vi "TAT-Create Reciepe.vi"(8 "Error In":errorcluster) -> (0 "error out":errorcluster)   [LabVIEW 2017]
uses:
  Controls/Recipe.ctl
  <vilib>/Utility/config.llb/Write Key (String).vi
  <vilib>/Utility/config.llb/Read Key (String).vi
  <vilib>/Utility/config.llb/NI_LVConfig.lvlib
panel:
  in  "Lable Data":T1
  in  "Reference Barcode":T2
  in  "T-Bin Seq. Select":T3 {"First" max=8 step=1; "Second" max=8 step=1; "Third" max=8 step=1; "Fourth" max=8 step=1; "Fifth" max=8 step=1; "Gun Enable" max=8}
  in  "Torquing Station Sensor Selection":T4
  in  "A-Bin Seq. Select":T5 {"Camera-2 Trig" max=8 step=1; "Camera-1 Trig" max=8 step=1; "First" max=8 step=1; "Second" max=8 step=1; "Third" max=8 step=1; "Fourth" max=8 step=1; "Fifth" max=8 step=1; "Sixth" max=8; "Seventh" max=8; "Eighth" max=8}
  in  "Ass. Sensor Select":T6 {"Gun \nProg. no." max=8 step=1; "Camera-2\n Prog. no." max=8 step=1; "Camera-1\n Prog. no." max=8 step=1}
  in  "Delete":bool
  in  "Save":bool
  in  "BACK":bool
  in  "PART NAME":string(combo)
  # "TEST PARAMETER SETTING"
  # "Bin No."
  # "Bin No."
  # "Bin No."
  # "Bin No."
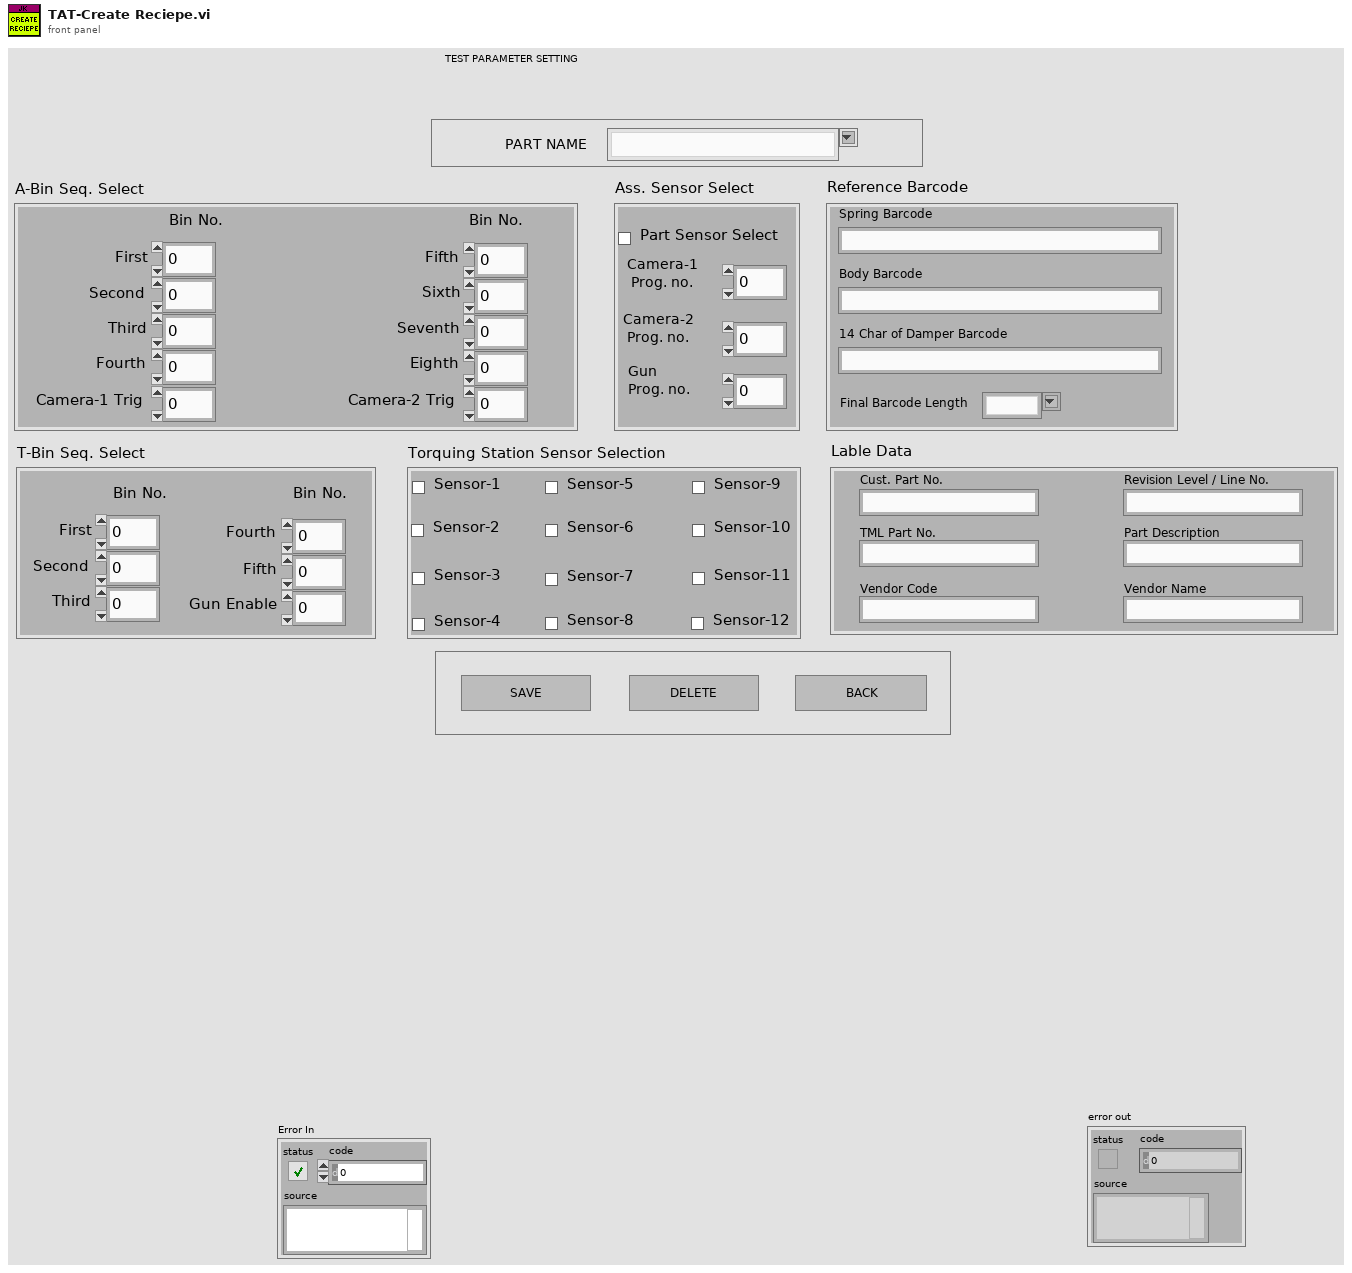
[diagram p1: front panel]
types:
  T1 = cluster{"Cust. Part No.":string, "TML Part No.":string, "Vendor Code":string, "Revision Level / Line No.":string, "Part Description":string, "Vendor Name":string}
  T2 = cluster{"Spring Barcode":string, "Body Barcode":string, "14 Char of Damper Barcode":string, "Final Barcode Length":string}
  T3 = cluster{"First":u16, "Second":u16, "Third":u16, "Fourth":u16, "Fifth":u16, "Gun Enable":u16}
  T4 = cluster{"Sensor-1":bool, "Sensor-2":bool, "Sensor-3":bool, "Sensor-4":bool, "Sensor-5":bool, "Sensor-6":bool, "Sensor-7":bool, "Sensor-8":bool, "Sensor-9":bool, "Sensor-10":bool, "Sensor-11":bool, "Sensor-12":bool}
  T5 = cluster{"First":u16, "Second":u16, "Third":u16, "Fourth":u16, "Fifth":u16, "Sixth":u16, "Seventh":u16, "Eighth":u16, "Camera-1 Trig":u16, "Camera-2 Trig":u16}
  T6 = cluster{"Part Sensor Select":bool, "Camera-1\n Prog. no.":u16, "Camera-2\n Prog. no.":u16, "Gun \nProg. no.":u16}
  T7 = enum32{"invalid app kind", "Development System", "Run Time System", "Student Edition", "Embedded LabVIEW", "Evaluation", "Custom"}
  T8 = typedef "NI_LVConfig.lvlib/Config Data RefNum.ctl" = refnum<k1>
  T9 = typedef "Recipe.ctl" = cluster{"Ass. Sensor Select":cluster{"Ass. Sensor Select":bool, "Camera-1 \nProg No.":u16, "Camera-2 \nProg No.":u16, "Gun \nProg No.":u16}, "Torque Sensor Select":cluster{"Torque Sensor-1":bool, "Torque Sensor-2":bool, "Torque Sensor-3":bool, "Torque Sensor-4":bool, "Torque Sensor-5":bool, "Torque Sensor-6":bool, "Torque Sensor-7":bool, "Torque Sensor-8":bool, "Torque Sensor-9":bool, "Torque Sensor-10":bool, "Torque Sensor-11":bool, "Torque Sensor-12":bool}, "Bin Seq. Select":cluster{"First Bin":u16, "Second Bin":u16, "Third Bin":u16, "Fourth Bin":u16, "Fifth Bin":u16, "Sixth Bin":u16, "Seventh Bin":u16, "Eighth Bin":u16, "Camera-1 Trig":u16, "Camera-2 Trig":u16}, "T-Bin Seq. Select":cluster{"First":u16, "Second":u16, "Third":u16, "Fourth":u16, "Fifth":u16, "Sixth":u16}, "Reference Barcode":cluster{"Spring Barcode":string, "Body Barcode":string, "14 Char of Barcode":string, "Final Barcode Length":string}, "Label Data":cluster{"Cust. Part No.":string, "TML Part No.":string, "Vendor Code":string, "Revision Level":string, "Part Description":string, "Vendor Name":string}}
  T10 = cluster{"First Bin":u16, "Second Bin":u16, "Third Bin":u16, "Fourth Bin":u16, "Fifth Bin":u16, "Sixth Bin":u16, "Seventh Bin":u16, "Eighth Bin":u16, "Camera-1 Trig":u16, "Camera-2 Trig":u16}
  T11 = cluster{"Ass. Sensor Select":bool, "Camera-1 \nProg No.":u16, "Camera-2 \nProg No.":u16, "Gun \nProg No.":u16}
  T12 = cluster{"Torque Sensor-1":bool, "Torque Sensor-2":bool, "Torque Sensor-3":bool, "Torque Sensor-4":bool, "Torque Sensor-5":bool, "Torque Sensor-6":bool, "Torque Sensor-7":bool, "Torque Sensor-8":bool, "Torque Sensor-9":bool, "Torque Sensor-10":bool, "Torque Sensor-11":bool, "Torque Sensor-12":bool}
  T13 = cluster{"First":u16, "Second":u16, "Third":u16, "Fourth":u16, "Fifth":u16, "Sixth":u16}
  T14 = cluster{"Spring Barcode":string, "Body Barcode":string, "14 Char of Barcode":string, "Final Barcode Length":string}
  T15 = cluster{"Cust. Part No.":string, "TML Part No.":string, "Vendor Code":string, "Revision Level":string, "Part Description":string, "Vendor Name":string}
  T16 = enum32{"Invalid", "Standard", "Closed", "Hidden", "Minimized", "Maximized"}
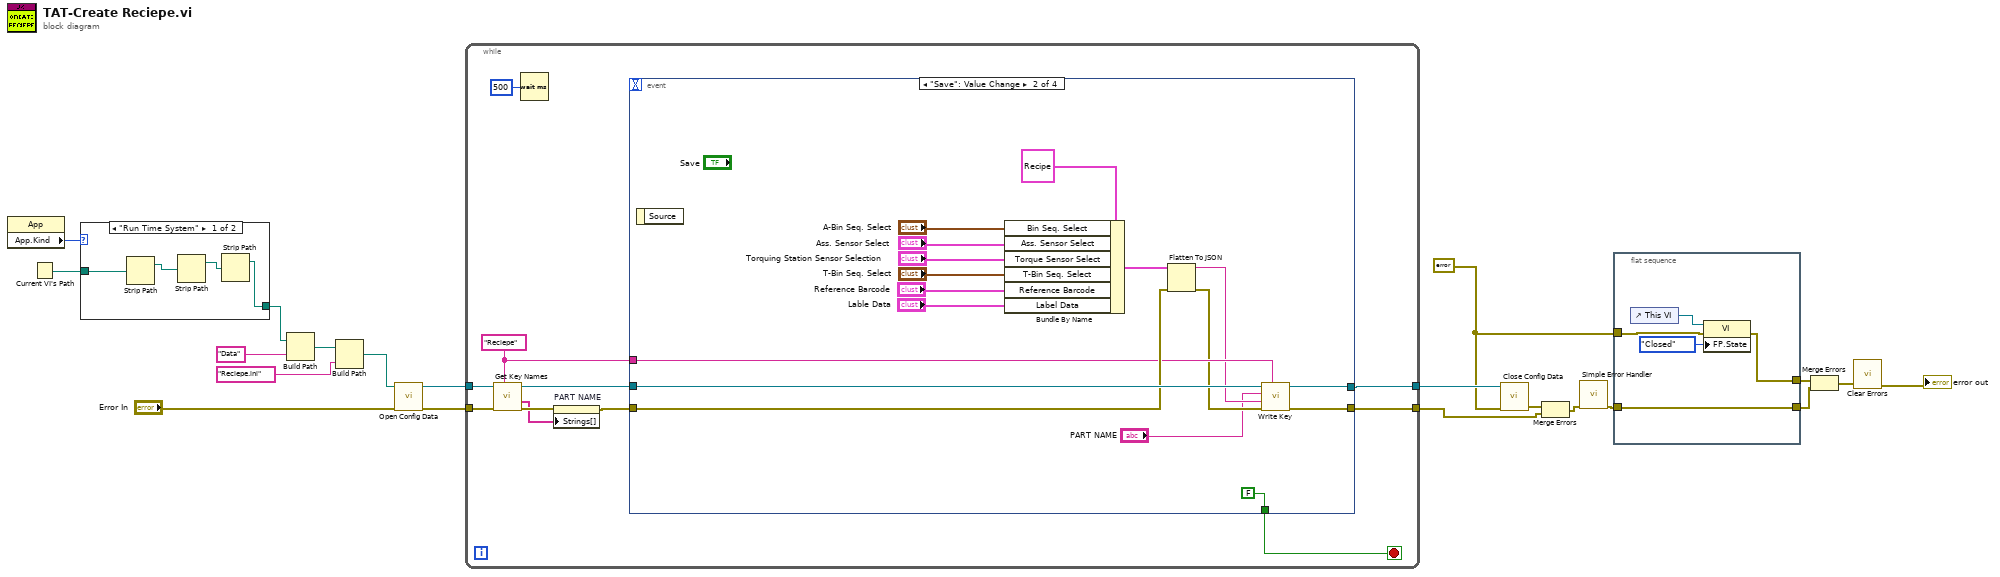
[diagram p0: block diagram]
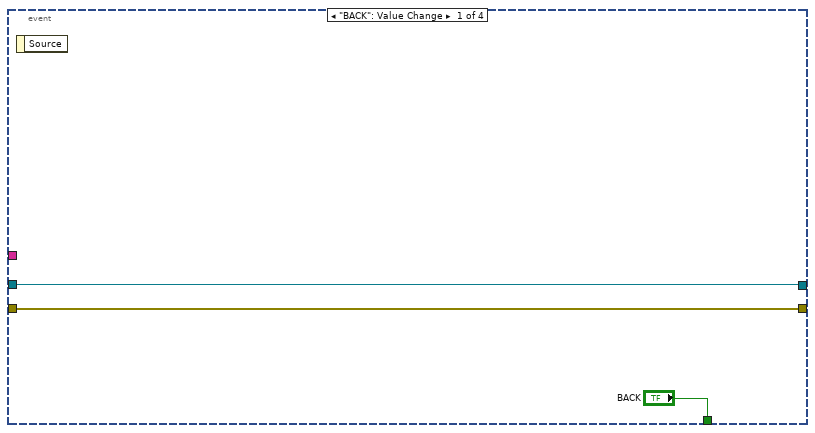
[diagram p2: hidden frame]
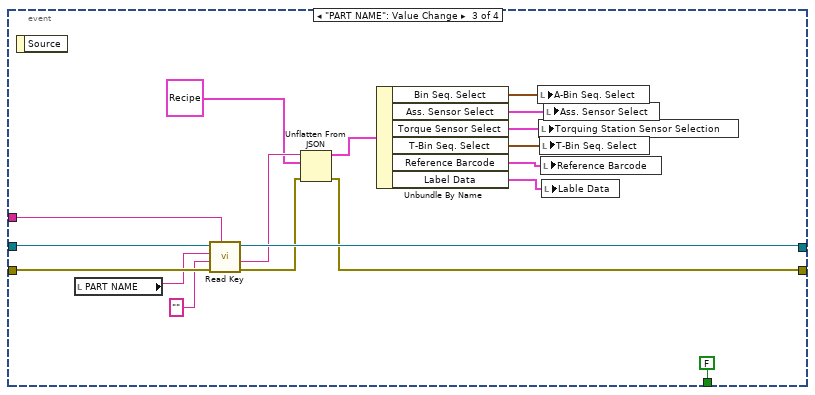
[diagram p3: hidden frame]
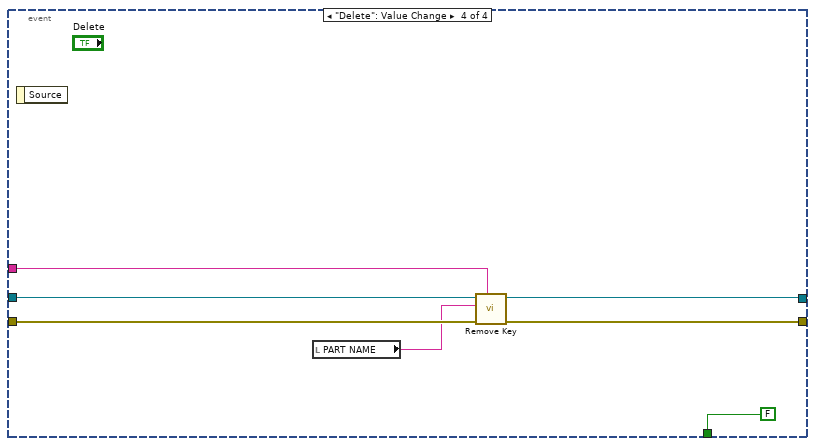
[diagram p4: hidden frame]
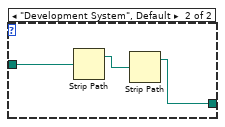
[diagram p5: hidden frame]
diagram:
  w4 = errorcluster {"status"=FALSE, "code"=0, "source"=""} ("error in (no error)")
  n1 = property class="App"() -> ("App.Kind"=w18:T7)  [unwired: 2 in, 2 out]
  n2 = Current VI's Path() -> (path=w19:path)
  n3 = case shown="\"Run Time System\"" w18 {
    tunnel: w19 -> [w22 w26]
    tunnel: [w21 w25] -> w16
    frame "Run Time System" {
      n4 = Strip Path(path=w22) -> (stripped path=w24:path)  [unwired: 1 out]
      n5 = Strip Path(path=w24) -> (stripped path=w23:path)  [unwired: 1 out]
      n6 = Strip Path(path=w23) -> (stripped path=w21:path)  [unwired: 1 out]
    }
    frame "Development System", Default {
      n7 = Strip Path(path=w26) -> (stripped path=w27:path)  [unwired: 1 out]
      n8 = Strip Path(path=w27) -> (stripped path=w25:path)  [unwired: 1 out]
    }
  }
  n9 = Build Path(base path=w16, name or relative path="Data") -> (appended path=w17:path)
  n10 = Build Path(base path=w17, name or relative path="Reciepe.ini") -> (appended path=w15:path)
  n11 = call <vilib>:"Open Config Data.vi"("error in (no error)"="Error In", "configuration file path"=w15) -> ("error out"=w3:errorcluster, "refnum"=w6:T8)  [unwired: 7 in, 1 out]
  n12 = while {
    tunnel: w6 -> [w34]
    tunnel: [w37] -> w5
    tunnel: [w36] -> w1
    tunnel: w3 -> [w35]
    stop <- w38 stop-if-true
    w32 = "Reciepe" ("section")
    n13 = call <vilib>:"Get Key Names.vi"("section"=w32, "error in (no error)"=w35, "refnum"=w34) -> ("error out"=w29:errorcluster, "key names"=w28:string[], "refnum out"=w33:T8)  [unwired: 5 in, 1 out]
    n14 = Wait (ms)(milliseconds to wait=u32 500) -> ()  [unwired: 1 out]
    n15 = property on="PART NAME" class="CmbBox"(error in=w29, "Strings[]"=w28) -> (error out=w30:errorcluster)  [unwired: 1 in, 1 out]
    n16 = event shown="[1] \"Save\": Value Change" {
      selector: _ -> [_ _ _ _]
      dyn-events: _ -> [_ _ _ _]
      timeout: _ -> [_ _ _ _]
      tunnel: ["BACK" FALSE ("BACK") FALSE ("BACK") FALSE ("BACK")] -> w38
      tunnel: [w40 w57 w72 w79] -> w37
      tunnel: w33 -> [w40 w58 w76 w80]
      tunnel: [w39 w56 w69 w81] -> w36
      tunnel: w30 -> [w39 w55 w75 w82]
      tunnel: w32 -> [_ w53 w74 w78]
      event "BACK": Value Change {
        n17 = event-data() -> ()  [unwired: 1 in, 1 out]
      }
      event "Save": Value Change {
        n18 = event-data() -> ()  [unwired: 1 in, 1 out]
        n19 = Bundle By Name(cluster=T9 {"Ass. Sensor Select"={"Ass. Sensor Select"=FALSE, "Camera-1 \nProg No."=0, "Camera-2 \nProg No."=0, "Gun \nProg No."=0}, "Torque Sensor Select"={"Torque Sensor-1"=FALSE, "Torque Sensor-2"=FALSE, "Torque Sensor-3"=FALSE, "Torque Sensor-4"=FALSE, "Torque Sensor-5"=FALSE, "Torque Sensor-6"=FALSE, "Torque Sensor-7"=FALSE, "Torque Sensor-8"=FALSE, "Torque Sensor-9"=FALSE, "Torque Sensor-10"=FALSE, "Torque Sensor-11"=FALSE, "Torque Sensor-12"=FALSE}, "Bin Seq. Select"={"First Bin"=0, "Second Bin"=0, "Third Bin"=0, "Fourth Bin"=0, "Fifth Bin"=0, "Sixth Bin"=0, "Seventh Bin"=0, "Eighth Bin"=0, "Camera-1 Trig"=0, "Camera-2 Trig"=0}, "T-Bin Seq. Select"={"First"=0, "Second"=0, "Third"=0, "Fourth"=0, "Fifth"=0, "Sixth"=0}, "Reference Barcode"={"Spring Barcode"="", "Body Barcode"="", "14 Char of Barcode"="", "Final Barcode Length"=""}, "Label Data"={"Cust. Part No."="", "TML Part No."="", "Vendor Code"="", "Revision Level"="", "Part Description"="", "Vendor Name"=""}}, "Bin Seq. Select"="A-Bin Seq. Select", "Ass. Sensor Select"="Ass. Sensor Select", "Torque Sensor Select"="Torquing Station Sensor Selection", "T-Bin Seq. Select"="T-Bin Seq. Select", "Reference Barcode"="Reference Barcode", "Label Data"="Lable Data") -> (w49:T9)
        n20 = Flatten To JSON(anything=w49, error in (no error)=w55) -> (JSON string=w47:string, 11:w48:errorcluster)  [unwired: 1 in]
        n21 = call-poly <vilib>:"Write Key.vi"("section"=w53, "error in (no error)"=w48, "value"=w47, "key"="PART NAME", "refnum"=w58) -> ("error out"=w56:errorcluster, "refnum out"=w57:T8)  [unwired: 4 in, 1 out]
      }
      event "PART NAME": Value Change {
        n22 = event-data() -> ()  [unwired: 1 in, 1 out]
        n23 = local read "PART NAME"() -> (w66:string)
        n24 = call-poly <vilib>:"Read Key.vi"("section"=w74, "error in (no error)"=w75, "default value"="", "key"=w66, "refnum"=w76) -> ("error out"=w70:errorcluster, "value"=w71:string, "refnum out"=w72:T8)  [unwired: 3 in, 1 out]
        n25 = Unflatten From JSON(JSON string=w71, type and defaults=T9 {"Ass. Sensor Select"={"Ass. Sensor Select"=FALSE, "Camera-1 \nProg No."=0, "Camera-2 \nProg No."=0, "Gun \nProg No."=0}, "Torque Sensor Select"={"Torque Sensor-1"=FALSE, "Torque Sensor-2"=FALSE, "Torque Sensor-3"=FALSE, "Torque Sensor-4"=FALSE, "Torque Sensor-5"=FALSE, "Torque Sensor-6"=FALSE, "Torque Sensor-7"=FALSE, "Torque Sensor-8"=FALSE, "Torque Sensor-9"=FALSE, "Torque Sensor-10"=FALSE, "Torque Sensor-11"=FALSE, "Torque Sensor-12"=FALSE}, "Bin Seq. Select"={"First Bin"=0, "Second Bin"=0, "Third Bin"=0, "Fourth Bin"=0, "Fifth Bin"=0, "Sixth Bin"=0, "Seventh Bin"=0, "Eighth Bin"=0, "Camera-1 Trig"=0, "Camera-2 Trig"=0}, "T-Bin Seq. Select"={"First"=0, "Second"=0, "Third"=0, "Fourth"=0, "Fifth"=0, "Sixth"=0}, "Reference Barcode"={"Spring Barcode"="", "Body Barcode"="", "14 Char of Barcode"="", "Final Barcode Length"=""}, "Label Data"={"Cust. Part No."="", "TML Part No."="", "Vendor Code"="", "Revision Level"="", "Part Description"="", "Vendor Name"=""}}, error in (no error)=w70) -> (value=w67:T9, error out=w69:errorcluster)  [unwired: 4 in]
        n26 = Unbundle By Name(w67) -> ("Bin Seq. Select"=w64:T10, "Ass. Sensor Select"=w63:T11, "Torque Sensor Select"=w62:T12, "T-Bin Seq. Select"=w61:T13, "Reference Barcode"=w60:T14, "Label Data"=w59:T15)
        n27 = local write "A-Bin Seq. Select"(w64) -> ()
        n28 = local write "Torquing Station Sensor Selection"(w62) -> ()
        n29 = local write "T-Bin Seq. Select"(w61) -> ()
        n30 = local write "Reference Barcode"(w60) -> ()
        n31 = local write "Lable Data"(w59) -> ()
        n32 = local write "Ass. Sensor Select"(w63) -> ()
      }
      event "Delete": Value Change {
        n33 = event-data() -> ()  [unwired: 1 in, 1 out]
        n34 = local read "PART NAME"() -> (w77:string)
        n35 = call <vilib>:"Remove Key.vi"("section"=w78, "error in (no error)"=w82, "key"=w77, "refnum"=w80) -> ("error out"=w81:errorcluster, "refnum out"=w79:T8)  [unwired: 5 in, 1 out]
      }
    }
  }
  n36 = call <vilib>:"Close Config Data.vi"("error in (no error)"=w4, "refnum"=w5) -> ("error out"=w12:errorcluster)  [unwired: 8 in, 1 out]
  n37 = Merge Errors(w12, w1) -> (w2:errorcluster)
  n38 = call <vilib>:"Simple Error Handler.vi"("error in (no error)"=w2) -> ("error out"=w7:errorcluster)  [unwired: 4 in, 4 out]
  n39 = flat-sequence {
    tunnel: w4 -> [w86]
    tunnel: [w85] -> w11
    tunnel: [w84] -> w8
    tunnel: w7 -> [w84]
    frame #0 {
      n40 = control-ref of="This VI"() -> (w88:refnum<vi>)
      n41 = property class="VI"(reference=w88, error in=w86, "FP.State"=T16."Closed" ("Front Panel Window:State")) -> (error out=w85:errorcluster)  [unwired: 1 out]
    }
  }
  n42 = Merge Errors(w11, w8) -> (w10:errorcluster)
  n43 = call <vilib>:"Clear Errors.vi"("error in (no error)"=w10) -> ("error out"=→"error out":errorcluster)  [unwired: 5 in, 1 out]
